vi "reg put process.vi"(11 "reg data in":T1(array[cluster])) -> (1 "room":string, 2 "reg data out":T1(array[cluster]), 3 "Array":bool[](array[boolean]))   [LabVIEW 2019]
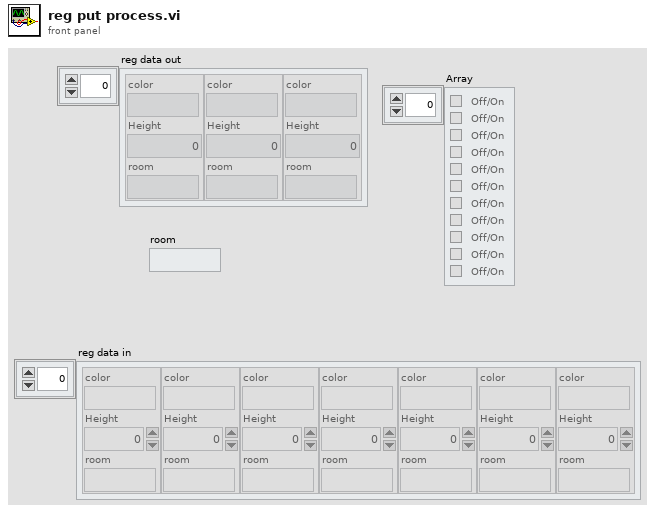
[diagram p1: front panel]
types:
  T1 = cluster{"color":string, "Height":i32, "room":string}[]
  T2 = cluster{"color":string, "Height":i32, "room":string}
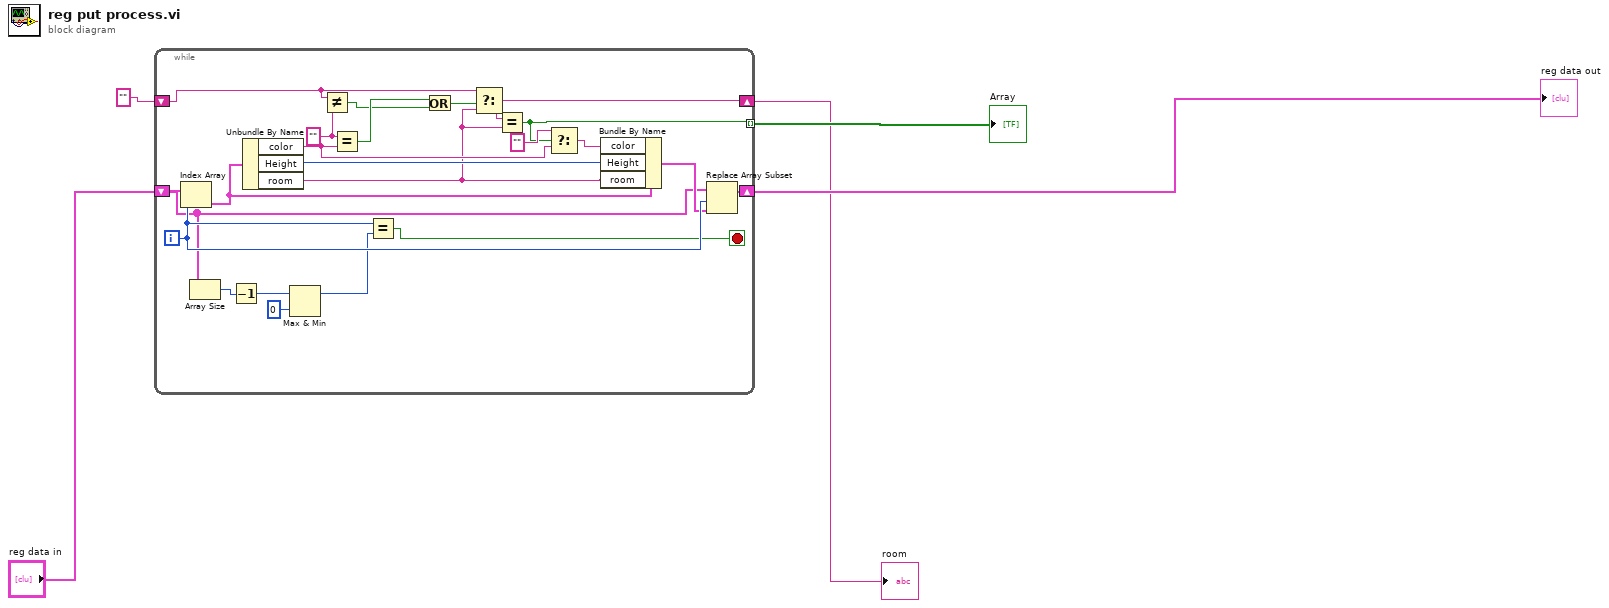
[diagram p0: block diagram]
diagram:
  n1 = while {
    shift-right: [w22] -> w5
    shift-left: "reg data in" -> [w10]
    shift-right: [w17] -> w3
    shift-left: "" -> [w25]
    tunnel: [w12] -> w4 mode=indexing
    i -> [w21]
    stop <- w11 stop-if-true
    w26 = "" ("x")
    n2 = Index Array(array=w10, index=w21) -> (element=w20:T2)
    n3 = Array Size(array=w10) -> (size(s)=w9:i32)
    n4 = Decrement(x=w9) -> (x-1=w8:i32)
    n5 = Unbundle By Name(w20) -> ("color"=w16:string, "Height"=w18:i32, "room"=w13:string)
    n6 = Max & Min(x=w8, y=0) -> (max(x,y)=w7:i32)  [unwired: 1 out]
    n7 = Not Equal?(x=w25, y=w26) -> (x != y?=w24:bool)
    n8 = Equal?(x=w26, y=w16) -> (x = y?=w27:bool)
    n9 = Equal?(x=w21, y=w7) -> (x = y?=w11:bool)
    n10 = Or(x=w27, y=w24) -> (x .or. y?=w23:bool)
    n11 = Select(t=w25, s=w23, f=w13) -> (s? t:f=w17:string)
    n12 = Equal?(x=w17, y=w13) -> (x = y?=w12:bool)
    n13 = Select(t="", s=w12, f=w16) -> (s? t:f=w15:string)
    n14 = Bundle By Name(cluster=w20, "color"=w15, "Height"=w18, "room"=w13) -> (w19:T2)
    n15 = Replace Array Subset(array=w10, new element=w19, index=w21) -> (w22:T1)
  }
  "reg data out" <- w5
  "Array" <- w4
  "room" <- w3
